vi "Get Detector.vi"(8 "error in (no error)":errorcluster, 10 "ypixels":i32, 11 "xpixels":i32) -> (0 "error out":errorcluster, 1 "function return":u32, 2 "ypixels out":i32, 3 "xpixels out":i32)   [LabVIEW 2014, in "atmcd32d.lvlib"]
doc: "unsigned int WINAPI GetDetector(int * xpixels, int * ypixels);"
uses:
  atmcd32d.lvlib
  atmcd32d.dll
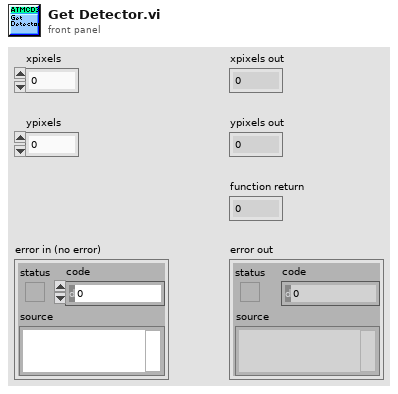
[diagram p1: front panel]
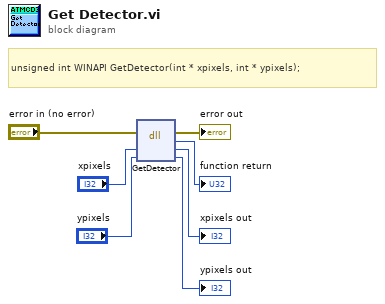
[diagram p0: block diagram]
diagram:
  # "unsigned int WINAPI GetDetector(int * xpixels, int * ypixels);"
  n1 = dll-call lib="C:/Users/Bakir/Documents/Lambda2-Testing/lib/Andorlib/atmcd32d.*" fn="GetDetector"(error in="error in (no error)", "xpixels"="xpixels", "ypixels"="ypixels") -> (error out=→"error out":errorcluster, →"function return":u32, "xpixels"=→"xpixels out":i32, "ypixels"=→"ypixels out":i32)  [unwired: 2 in, 1 out]
